vi "test2-LocalExternalStatusRegistrationViaAPI.vi"(8 "error in (no error)":errorcluster, 11 "TestCase in":refnum<class "testcase-CSMBroadcast.lvclass">) -> (0 "error out":errorcluster, 3 "TestCase out":refnum<class "testcase-CSMBroadcast.lvclass">)   [LabVIEW 2017, in "testcase-CSMBroadcast.lvclass"]
uses:
  testcase-CSMBroadcast.lvclass
  0b17d103-e67b-41be-a9eb-a2ee1311ff1f.vi
  5999693e-4f8a-4b34-ae87-f34dff5771be.vi
  52a2a10a-a04b-4bad-8df4-e1eb944f47cc.vi
  826f03dd-b4b5-4c6b-9085-8edf6da4f43b.vi
  src/user.lib/_NEVSTOP/Communicable State Machine(CSM)/AdvanceAPI/CSM - Get Module Attribute.vi
  <vilib>/addons/_JKI Toolkits/VI Tester/TestCase.llb/TestCase.lvclass
  src/user.lib/_NEVSTOP/Communicable State Machine(CSM)/Communicable State Machine.lvlib
  CSM/CSM-Testcase.lvlib
  C:/Program Files (x86)/National Instruments/LabVIEW 2017/vi.lib/addons/_JKI Toolkits/VI Tester/TestCase.llb/TestCase.lvclass
panel:
  out "LoopCount 2":i32
  out "LoopCount":i32
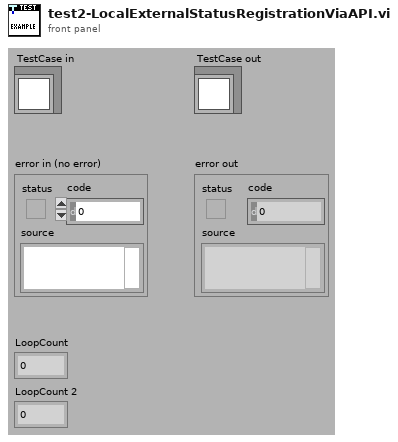
[diagram p1: front panel]
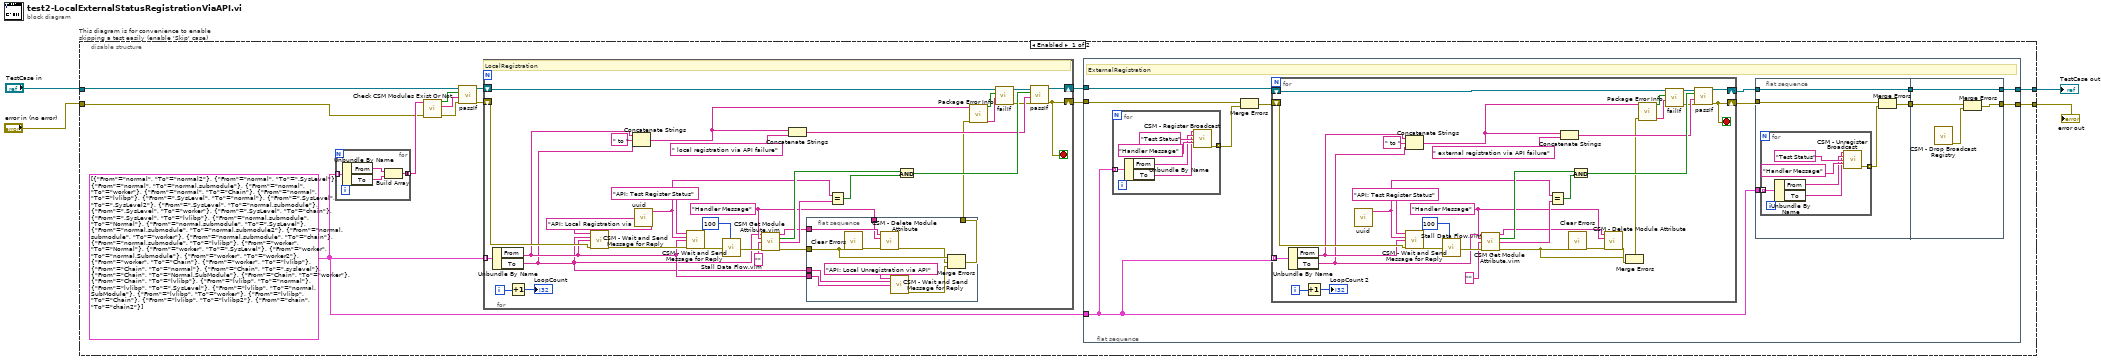
[diagram p0: block diagram]
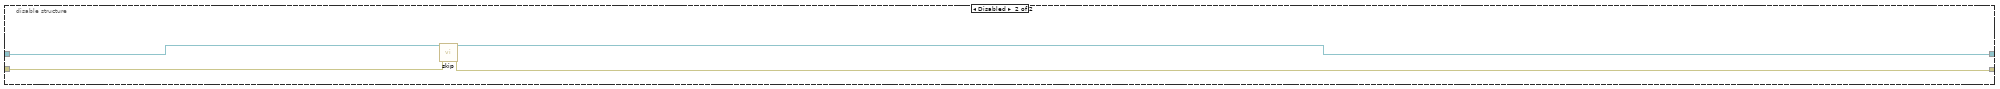
[diagram p2: hidden frame]
diagram:
  n1 = disable-structure "This diagram is for convenience to enable skipping a test easily (enable 'Skip' case)" shown="Enabled" {
    disable-tunnel: "TestCase in" -> [w11 w133]
    disable-tunnel: [w6 w131] -> w1
    disable-tunnel: [w5 w132] -> w3
    disable-tunnel: "error in (no error)" -> [w9 w130]
    frame Enabled {
      w7 = cluster{"From":string, "To":string}[] [{"From"="normal", "To"="normal2"}, {"From"="normal", "To"=".SysLevel"}, {"From"="normal", "To"="normal.submodule"}, {"From"="normal", "To"="worker"}, {"From"="normal", "To"="Chain"}, {"From"="normal", "To"="lvlibp"}, {"From"=".SysLevel", "To"="normal"}, {"From"=".SysLevel", "To"=".SysLevel2"}, {"From"=".SysLevel", "To"="normal.submodule"}, {"From"=".SysLevel", "To"="worker"}, {"From"=".SysLevel", "To"="chain"}, {"From"=".SysLevel", "To"="lvlibp"}, {"From"="normal.submodule", "To"="Normal"}, {"From"="normal.submodule", "To"=".SysLevel"}, {"From"="normal.submodule", "To"="normal.submodule2"}, {"From"="normal.submodule", "To"="worker"}, {"From"="normal.submodule", "To"="chain"}, {"From"="normal.submodule", "To"="lvlibp"}, {"From"="worker", "To"="Normal"}, {"From"="worker", "To"=".SysLevel"}, {"From"="worker", "To"="normal.Submodule"}, {"From"="worker", "To"="worker2"}, {"From"="worker", "To"="Chain"}, {"From"="worker", "To"="lvlibp"}, {"From"="Chain", "To"="normal"}, {"From"="Chain", "To"=".syslevel"}, {"From"="Chain", "To"="Normal.SubModule"}, {"From"="Chain", "To"="worker"}, {"From"="Chain", "To"="lvlibp"}, {"From"="lvlibp", "To"="normal"}, {"From"="lvlibp", "To"=".SysLevel"}, {"From"="lvlibp", "To"="normal.SubModule"}, {"From"="lvlibp", "To"="worker"}, {"From"="lvlibp", "To"="Chain"}, {"From"="lvlibp", "To"="lvlibp2"}, {"From"="chain", "To"="chain2"}]
      n2 = for {
        tunnel: w7 -> [w21] mode=indexing
        tunnel: [w18] -> w14 mode=concatenating
        n3 = Unbundle By Name(w21) -> ("From"=w20:string, "To"=w19:string)
        n4 = Build Array(w20, w19) -> (w18:string[])
      }
      n5 = call "Check CSM Modules Exist Or Not.vi"("error in"=w9, "CSM names in"=w14) -> ("error out"=w12:errorcluster, "Debug string"=w13:string, "All Modules Exist?"=w15:bool)  [unwired: 7 in]
      n6 = call-dynamic "passIf.vi"("error in (no error)"=w12, "message (\"\")"=w13, "pass"=w15, "TestCase in"=w11) -> ("error out"=w8:errorcluster, "TestCase out"=w10:refnum<class "testcase-CSMBroadcast.lvclass">)  [unwired: 6 in]
      n7 = for {
        shift-right: [w34] -> w16
        shift-left: w8 -> [w35]
        shift-right: [w41] -> w17
        shift-left: w10 -> [w26]
        tunnel: w7 -> [w52] mode=indexing
        i -> [w54]
        stop <- w34 stop-if-true
        w36 = "Handler Message" ("To")
        # "LocalRegistration"
        n8 = Unbundle By Name(w52) -> ("From"=w31:string, "To"=w30:string)
        n9 = Increment(x=w54) -> (x+1=→"LoopCount":i32)
        n10 = call "CSM - Wait and Send Message for Reply.vi"("State"="API: Local Registration via API", "Arguments (\"\")"=w30, "Target Module"=w31, "Error In (No Error)"=w35) -> ("error out"=w49:errorcluster)  [unwired: 8 in, 3 out]
        n11 = Concatenate Strings(w31, " to " ("string"), w30) -> (w22:string)
        n12 = call "uuid.vi"() -> ("UUID"=w43:string)  [unwired: 11 in]
        n13 = call "CSM - Wait and Send Message for Reply.vi"("State"="API: Test Register Status", "Arguments (\"\")"=w43, "Target Module"=w31, "Error In (No Error)"=w49) -> ("error out"=w48:errorcluster)  [unwired: 8 in, 3 out]
        n14 = call "Stall Data Flow.vim"("value in"=w48, "milliseconds to wait"=u32 100) -> ("value out"=w46:errorcluster)  [unwired: 1 out]
        n15 = call "CSM Get Module Attribute.vim"("CSM Name"=w30, "Attribute"=w36, "Default Value (Empty Variant)"="", "Error In"=w46) -> ("CSM Name (Dup)"=w37:string, "Found"=w45:bool, "Value"=w42:string, "error out"=w38:errorcluster)  [unwired: 7 in, 1 out]
        n16 = Concatenate Strings(w22, " local registration via API failure" ("string")) -> (w29:string)
        n17 = flat-sequence {
          tunnel: w38 -> [w58]
          tunnel: w37 -> [w63]
          tunnel: w36 -> [w62]
          tunnel: w30 -> [w60]
          tunnel: w31 -> [w59]
          tunnel: [w55] -> _
          tunnel: [w55] -> w23
          frame #0 {
            n18 = call <vilib>:"Clear Errors.vi"("error in (no error)"=w58) -> ("error out"=w64:errorcluster)  [unwired: 5 in, 1 out]
            n19 = call "CSM - Delete Module Attribute.vi"("CSM Name"=w63, "Attribute"=w62, "Error In"=w64) -> ("error out"=w57:errorcluster)  [unwired: 9 in, 3 out]
            n20 = call "CSM - Wait and Send Message for Reply.vi"("State"="API: Local Unregistration via API", "Arguments (\"\")"=w60, "Target Module"=w59) -> ("error out"=w56:errorcluster)  [unwired: 9 in, 3 out]
            n21 = Merge Errors(w58, w57, w56) -> (w55:errorcluster)
          }
        }
        n22 = Equal?(x=w43, y=w42) -> (x = y?=w40:bool)
        n23 = And(x=w45, y=w40) -> (x .and. y?=w39:bool)
        n24 = call "Package Error Info.vi"("error in"=w23, "String in"=w22) -> ("packed error info out"=w27:string, "error status"=w28:bool)  [unwired: 8 in]
        n25 = call-dynamic "failIf.vi"("message (\"\")"=w27, "fail"=w28, "TestCase in"=w26) -> ("error out"=w24:errorcluster, "TestCase out"=w25:refnum<class "testcase-CSMBroadcast.lvclass">)  [unwired: 7 in]
        n26 = call-dynamic "passIf.vi"("error in (no error)"=w24, "message (\"\")"=w29, "pass"=w39, "TestCase in"=w25) -> ("error out"=w34:errorcluster, "TestCase out"=w41:refnum<class "testcase-CSMBroadcast.lvclass">)  [unwired: 6 in]
      }
      n27 = flat-sequence {
        tunnel: w17 -> [w75]
        tunnel: w16 -> [w73]
        tunnel: w7 -> [w72]
        tunnel: [w66] -> w6
        tunnel: [w65] -> w5
        frame #0 {
          # "ExternalRegistration"
          n28 = for {
            tunnel: w72 -> [w96] mode=indexing
            tunnel: [w91] -> w71 mode=indexing
            n29 = Unbundle By Name(w96) -> ("From"=w93:string, "To"=w92:string)
            n30 = call "CSM - Register Broadcast.vi"("CSM Name(Empty for Broadcast Event)"=w92, "Source CSM Name (* as Default)"=w93, "Trigger"="Test Status" ("Status"), "API (If \"\", Same as Trigger)"="Handler Message" ("Response Message (If \"\", Same as Source Message)")) -> ("error out"=w91:errorcluster)  [unwired: 10 in, 1 out]
          }
          n31 = Merge Errors(w73, w71) -> (w74:errorcluster)
          n32 = for {
            shift-right: [w111] -> w70
            shift-left: w74 -> [w112]
            shift-right: [w118] -> w69
            shift-left: w75 -> [w101]
            tunnel: w72 -> [w127] mode=indexing
            i -> [w129]
            stop <- w111 stop-if-true
            w113 = "Handler Message" ("To")
            n33 = Unbundle By Name(w127) -> ("From"=w106:string, "To"=w105:string)
            n34 = Increment(x=w129) -> (x+1=→"LoopCount 2":i32)
            n35 = call "uuid.vi"() -> ("UUID"=w120:string)  [unwired: 11 in]
            n36 = Concatenate Strings(w106, " to " ("string"), w105) -> (w97:string)
            n37 = call "CSM - Wait and Send Message for Reply.vi"("State"="API: Test Register Status", "Arguments (\"\")"=w120, "Target Module"=w106, "Error In (No Error)"=w112) -> ("error out"=w125:errorcluster)  [unwired: 8 in, 3 out]
            n38 = call "Stall Data Flow.vim"("value in"=w125, "milliseconds to wait"=u32 100) -> ("value out"=w123:errorcluster)  [unwired: 1 out]
            n39 = call "CSM Get Module Attribute.vim"("CSM Name"=w105, "Attribute"=w113, "Default Value (Empty Variant)"="", "Error In"=w123) -> ("CSM Name (Dup)"=w114:string, "Found"=w122:bool, "Value"=w119:string, "error out"=w109:errorcluster)  [unwired: 7 in, 1 out]
            n40 = Equal?(x=w120, y=w119) -> (x = y?=w117:bool)
            n41 = Concatenate Strings(w97, " external registration via API failure" ("string")) -> (w104:string)
            n42 = call <vilib>:"Clear Errors.vi"("error in (no error)"=w109) -> ("error out"=w115:errorcluster)  [unwired: 5 in, 1 out]
            n43 = And(x=w122, y=w117) -> (x .and. y?=w116:bool)
            n44 = call "CSM - Delete Module Attribute.vi"("CSM Name"=w114, "Attribute"=w113, "Error In"=w115) -> ("error out"=w110:errorcluster)  [unwired: 9 in, 3 out]
            n45 = Merge Errors(w109, w110) -> (w98:errorcluster)
            n46 = call "Package Error Info.vi"("error in"=w98, "String in"=w97) -> ("packed error info out"=w102:string, "error status"=w103:bool)  [unwired: 8 in]
            n47 = call-dynamic "failIf.vi"("message (\"\")"=w102, "fail"=w103, "TestCase in"=w101) -> ("error out"=w99:errorcluster, "TestCase out"=w100:refnum<class "testcase-CSMBroadcast.lvclass">)  [unwired: 7 in]
            n48 = call-dynamic "passIf.vi"("error in (no error)"=w99, "message (\"\")"=w104, "pass"=w116, "TestCase in"=w100) -> ("error out"=w111:errorcluster, "TestCase out"=w118:refnum<class "testcase-CSMBroadcast.lvclass">)  [unwired: 6 in]
          }
          n49 = flat-sequence {
            tunnel: w72 -> [w80]
            tunnel: w70 -> [w78]
            tunnel: w69 -> [w79]
            tunnel: [w79] -> w68
            tunnel: [w76] -> w67
            tunnel: [w88] -> w65
            tunnel: [w90] -> w66
            tunnel: w68 -> [w90]
            tunnel: w67 -> [w89]
            frame #0 {
              n50 = for {
                tunnel: w80 -> [w86] mode=indexing
                tunnel: [w81] -> w77 mode=indexing
                n51 = Unbundle By Name(w86) -> ("From"=w83:string, "To"=w82:string)
                n52 = call "CSM - Unregister Broadcast.vi"("CSM Name(Empty for Broadcast Event)"=w82, "Source CSM Name (* as Default)"=w83, "Trigger"="Test Status" ("Status"), "API (\"*\" as Default)"="Handler Message" ("Response Message (If \"\", Same as Source Message)")) -> ("error out"=w81:errorcluster)  [unwired: 10 in, 1 out]
              }
              n53 = Merge Errors(w78, w77) -> (w76:errorcluster)
            }
            frame #1 {
              n54 = call "CSM - Drop Broadcast Registry.vi"() -> ("error out"=w87:errorcluster)  [unwired: 15 in]
              n55 = Merge Errors(w89, w87) -> (w88:errorcluster)
            }
          }
        }
      }
    }
    frame Disabled {
      # "skip test result while test is under development"
      n56 = call <vilib>:"skip.vi"("error in (no error)"=w130, "TestCase in"=w133) -> ("error out"=w132:errorcluster, "TestCase out"=w131:refnum<class "testcase-CSMBroadcast.lvclass">)  [unwired: 8 in]
    }
  }
  "error out" <- w3
  "TestCase out" <- w1
